vi "MagazineLogicTest.vi"() -> ()   [LabVIEW 2020]
panel:
  in  "Kicker Power":dbl
  in  "Magazine Power":dbl
  in  "Input Power":dbl
  out "Kicker Motors":dbl
  out "Magazine Motors":dbl
  out "Intake Motors":dbl
  out "Current State":T1(ring)
  in  "Initial State":T1(ring)
  in  "Outtake Side Sensor":bool
  in  "Intake Side Sensor":bool
  in  "Outtake Button":bool
  in  "Intake Toggle":bool
  # "Inputs"
  # "Power Levels"
  # "Outputs"
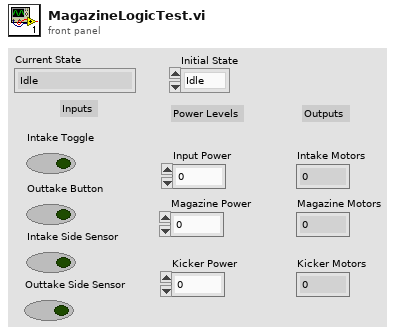
[diagram p1: front panel]
types:
  T1 = enum16{"Idle", "Waiting For Cargo", "Move Cargo", "Outtake"}
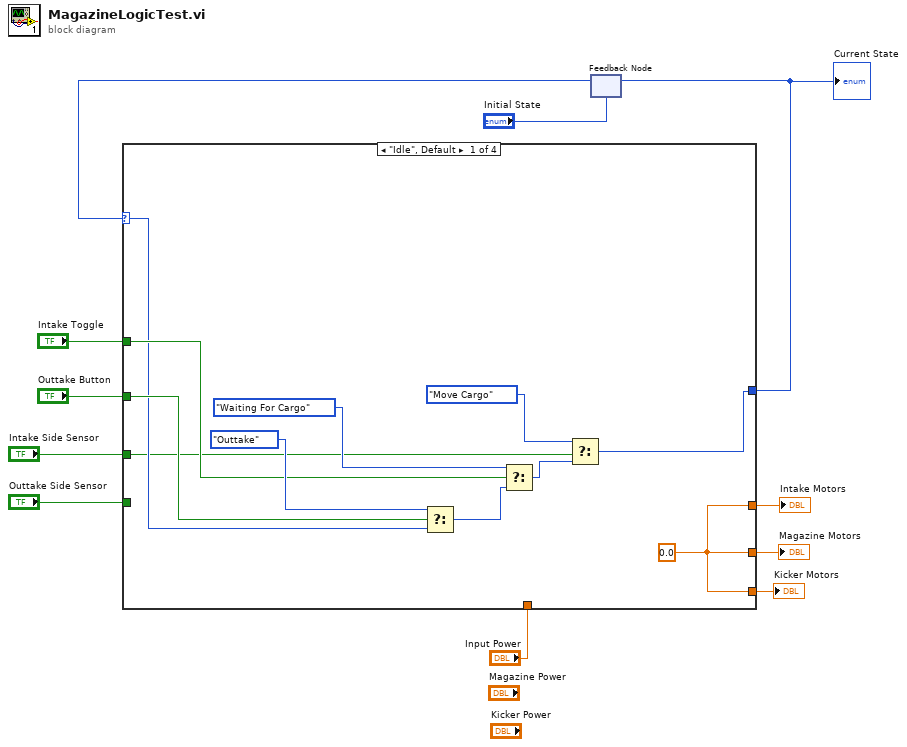
[diagram p0: block diagram]
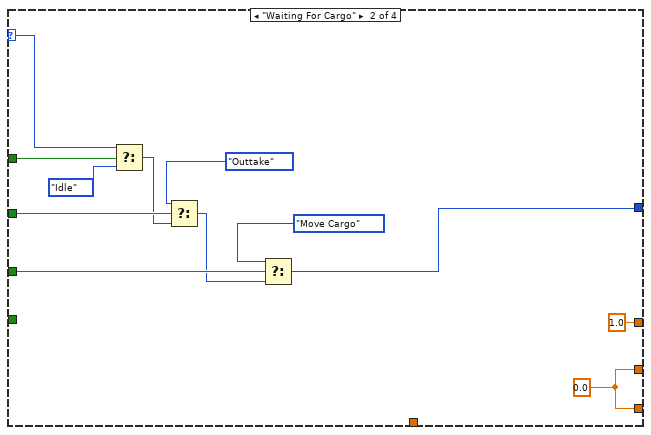
[diagram p2: hidden frame]
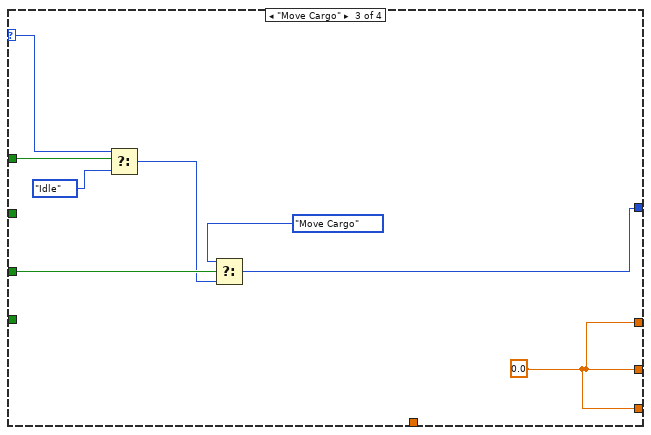
[diagram p3: hidden frame]
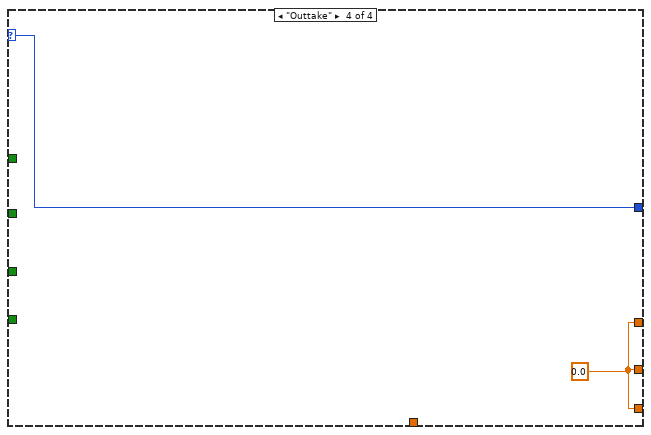
[diagram p4: hidden frame]
diagram:
  n1 = feedback #1("Initial State") -> (w10:T1)
  n2 = case shown="\"Idle\", Default" w10 {
    selector: w10 -> [w17 w29 w40 w44]
    tunnel: "Outtake Button" -> [w18 w27 _ _]
    tunnel: "Intake Toggle" -> [w19 w30 w41 _]
    tunnel: [w14 w33 w35 w44] -> w7
    tunnel: "Intake Side Sensor" -> [w13 w34 w38 _]
    tunnel: "Input Power" -> [_ _ _ _]
    tunnel: [w16 1.0 w42 w43] -> w4
    tunnel: [w16 w31 w42 w43] -> w3
    tunnel: [w16 w31 w42 w43] -> w2
    tunnel: "Outtake Side Sensor" -> [_ _ _ _]
    frame "Idle", Default {
      w16 = 0.0
      n3 = Select(t=T1."Outtake" ("Initial State"), s=w18, f=w17) -> (s? t:f=w22:T1)
      n4 = Select(t=T1."Waiting For Cargo" ("Initial State"), s=w19, f=w22) -> (s? t:f=w15:T1)
      n5 = Select(t=T1."Move Cargo" ("Initial State"), s=w13, f=w15) -> (s? t:f=w14:T1)
    }
    frame "Waiting For Cargo" {
      w31 = 0.0
      n6 = Select(t=w29, s=w30, f=T1."Idle" ("Initial State")) -> (s? t:f=w26:T1)
      n7 = Select(t=T1."Outtake" ("Initial State"), s=w27, f=w26) -> (s? t:f=w25:T1)
      n8 = Select(t=T1."Move Cargo" ("Initial State"), s=w34, f=w25) -> (s? t:f=w33:T1)
    }
    frame "Move Cargo" {
      w42 = 0.0
      n9 = Select(t=w40, s=w41, f=T1."Idle" ("Initial State")) -> (s? t:f=w37:T1)
      n10 = Select(t=T1."Move Cargo" ("Initial State"), s=w38, f=w37) -> (s? t:f=w35:T1)
    }
    frame "Outtake" {
      w43 = 0.0
    }
  }
  "Current State" <- w7
  "Intake Motors" <- w4
  "Magazine Motors" <- w3
  "Kicker Motors" <- w2
  n11 = feedback-in #1(w7) -> ()
